vi "Returning Values By Reference String Corrected.vi"(8 "error in (no error)":errorcluster, 11 "str":string) -> (0 "error out":errorcluster, 2 "newString out":string)   [LabVIEW 2009, in "LabVIEWWrapper_PassingDataSampleDLL.lvlib"]
doc: "void ReturningValuesByReference_String (char *str, char **newString);"
uses:
  LabVIEWWrapper_PassingDataSampleDLL.lvlib
  <vilib>/Utility/importsl/GetValueByPointer/GetValueByPointer.xnode
  <vilib>/Utility/importsl/GetValueByPointer/datatype.ctl
  Program Files (x86)/National Instruments/LabVIEW 2009/resource/lvimptsl.dll
  PassingDataSampleDLL.dll
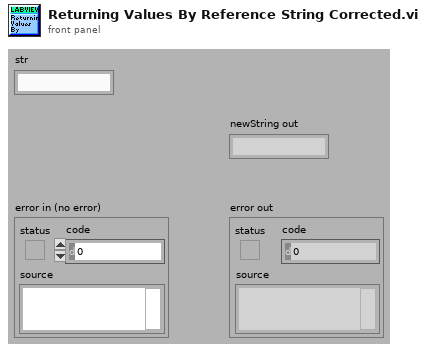
[diagram p1: front panel]
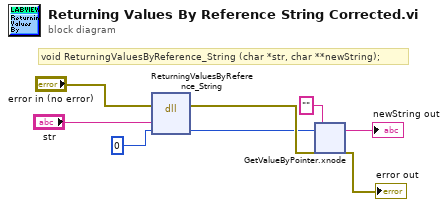
[diagram p0: block diagram]
diagram:
  # "void ReturningValuesByReference_String (char *str, char **newString);"
  n1 = dll-call lib="C:/My Dropbox/Systems Engineering Application/SDK/C Integration/LabVIEWWrapper/PassingDataSampleDLL.*" fn="ReturningValuesByReference_String"(error in="error in (no error)", "str"="str", "newString"=i64 0) -> (error out=w5:errorcluster, "newString"=w4:i64)  [unwired: 4 in, 1 out]
  n2 = xnode "GetValueByPointer.xnode"("Pointer"=w4, "InputType"="", "ErrorIn"=w5) -> ("Output"=→"newString out":string, "ErrorOut"=→"error out":errorcluster)  [unwired: 1 in]
